vi "Example_BoardSerialization.vi"() -> ()   [LabVIEW 2015, in "TronviewGame.lvlib" / "Board.lvclass"]
uses:
  Board.lvclass
  BoardSize.ctl
  Board.lvclass/Board.ctl
  GetBoard.vi
panel:
  out "Eq?":bool
  out "SerializedBoard":string
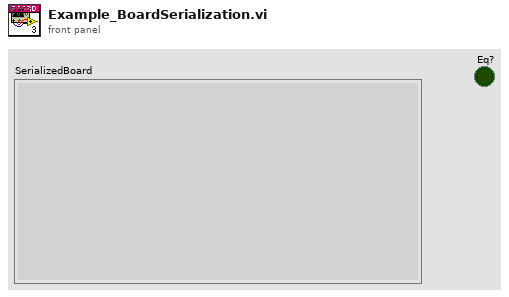
[diagram p1: front panel]
types:
  T1 = typedef "TronviewGame.lvlib/Board.lvclass/BoardSize.ctl" = cluster{"Columns":u16, "Rows":u16}
  T2 = typedef "TronviewGame.lvlib/Board.lvclass/FieldState.ctl" = enum16{"Empty", "Blocked", "Player1Position", "Player2Postion", "Player1Marked", "Player2Marked"}
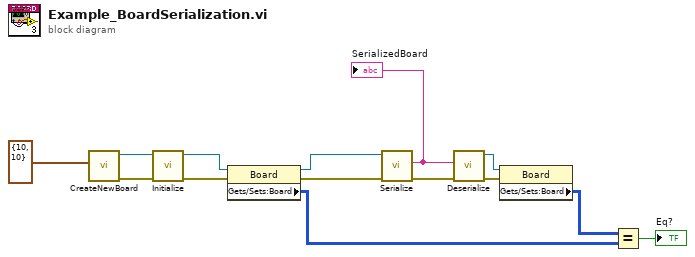
[diagram p0: block diagram]
diagram:
  n1 = call "CreateNewBoard.vi"("Size"=T1 {"Columns"=10, "Rows"=10}) -> ("error out"=w14:errorcluster, "Board out"=w13:refnum<class "Board.lvclass">)  [unwired: 9 in]
  n2 = call "Initialize.vi"("error in (no error)"=w14, "Board in"=w13) -> ("error out"=w12:errorcluster, "Board out"=w7:refnum<class "Board.lvclass">)  [unwired: 8 in]
  n3 = property class="Board"(reference=w7, error in=w12) -> (reference out=w6:refnum<class "Board.lvclass">, error out=w8:errorcluster, "Gets/Sets:Board"=w2:T2[][])
  n4 = call "Serialize.vi"("error in (no error)"=w8, "Board in"=w6) -> ("error out"=w10:errorcluster, "SerializedBoard"=w9:string)  [unwired: 7 in, 1 out]
  "SerializedBoard" <- w9
  n5 = call "Deserialize.vi"("error in (no error)"=w10, "SerializedBoard"=w9) -> ("error out"=w5:errorcluster, "Board out"=w4:refnum<class "Board.lvclass">)  [unwired: 8 in]
  n6 = property class="Board"(reference=w4, error in=w5) -> ("Gets/Sets:Board"=w3:T2[][])  [unwired: 2 out]
  n7 = Equal?(x=w3, y=w2) -> (x = y?=→"Eq?":bool)
